vi "PLC Project.vi"() -> ()   [LabVIEW 2022 SP3]
uses:
  <vilib>/MakerHub/LINX/Public/Peripherals/Digital/Digital Read 1 Chan.vi
  <vilib>/MakerHub/LINX/Public/Peripherals/PWM/PWM Set Duty Cycle 1 Chan.vi
  <vilib>/MakerHub/LINX/Public/Peripherals/Digital/Digital Write 1 Chan.vi
  <vilib>/MakerHub/LINX/Public/Peripherals/Digital/Digital Read N Chans.vi
  <vilib>/MakerHub/LINX/Public/Peripherals/Digital/Digital Write N Chans.vi
  <vilib>/MakerHub/LINX/Private/Local IO/LinxDigitalRead.vi
  <vilib>/MakerHub/LINX/Public/Utilities/Check Channel.vi
  <vilib>/MakerHub/LINX/Private/Local IO/LinxDigitalWrite.vi
  <vilib>/MakerHub/LINX/Public/Utilities/Open Serial.vi
  <vilib>/MakerHub/LINX/Private/Utilties/Generate Error.vi
  <vilib>/MakerHub/LINX/Public/Peripherals/PWM/PWM Set Duty Cycle N Chans.vi
  <vilib>/MakerHub/LINX/LMH-LINX.lvlib
  <vilib>/MakerHub/LINX/Public/Sensors/Distance/Ultrasonic/Ultrasonic.lvlib
panel:
  out "Centimeters":dbl
  out "Right":bool
  out "Left":bool
  in  "stop":bool
  in  "PWM signal  (0-255)":dbl
  in  "Input 1":bool
  in  "Input 3":bool
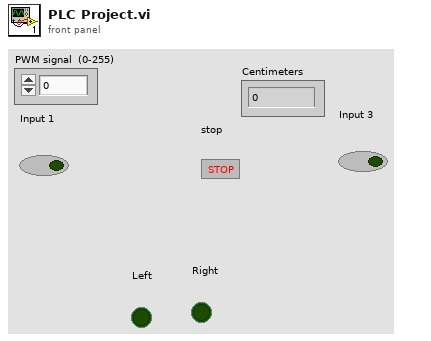
[diagram p1: front panel]
types:
  T1 = typedef "LMH-LINX.lvlib/LINX Ref.ctl" = cluster{"IO":T2, "Interface":T3, "LINX Device Config":T4}
  T2 = typedef "LMH-LINX.lvlib/Platform.ctl" = enum16{"Remote", "Local"}
  T3 = typedef "LMH-LINX.lvlib/Interface.ctl" = enum16{"Serial", "TCP"}
  T4 = typedef "LMH-LINX.lvlib/Device.lvlib/LINX Device Config.ctl" = cluster{"Interface":T3, "COM Port":refnum<visa-resource-name>, "TCP Configuration":T5, "Device Family":u8, "Device ID":u8, "Device Name":string, "TCP Ref":refnum<k5>, "Channels":T6}
  T5 = typedef "LMH-LINX.lvlib/Device.lvlib/TCP Config.ctl" = cluster{"IP Address":string, "Port":u16}
  T6 = typedef "LMH-LINX.lvlib/Channels.ctl" = cluster{"DI":u8[], "DO":u8[], "AI":u8[], "AO":u8[], "PWM":u8[], "QE":u8[], "UART":u8[], "I2C 2":u8[], "SPI":u8[], "CAN":u8[], "Servo":u8[], "AI Ref (V)":dbl, "AI Resolution (Bits)":u8, "AO Ref (V)":dbl, "AO Resolution (Bits)":u8}
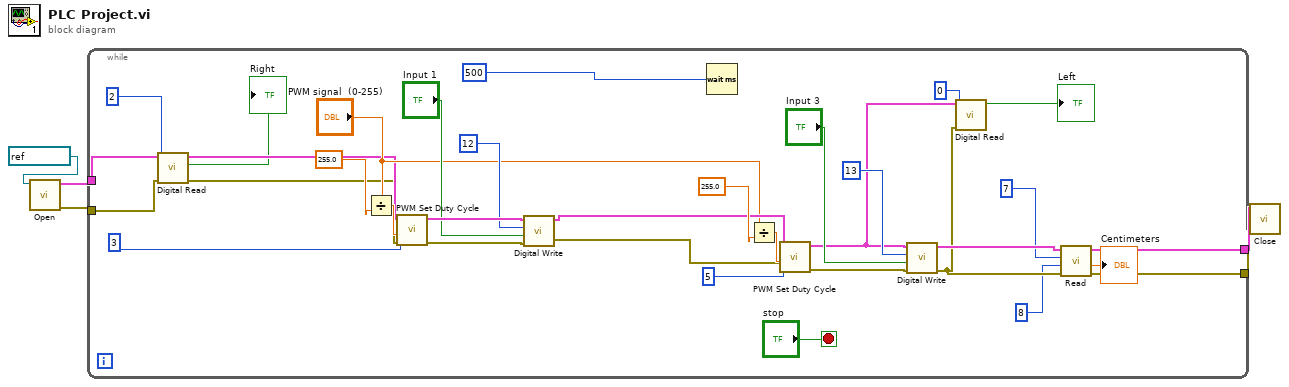
[diagram p0: block diagram]
diagram:
  n1 = call-poly <vilib>:"Open.vi"("Serial Port"=refnum<visa-resource-name> "COM5") -> ("Error Out"=w3:errorcluster, "LINX Resource"=w4:T1)  [unwired: 8 in, 1 out]
  n2 = while {
    tunnel: w4 -> [w21]
    tunnel: w3 -> [w19]
    tunnel: [w10] -> w2
    tunnel: [w9] -> w1
    stop <- "stop" stop-if-true
    n3 = call-poly <vilib>:"Digital Read.vi"("Error In"=w19, "DI Channel"=u8 2, "LINX Resource"=w21) -> ("Error Out"=w17:errorcluster, "DI Value"=→"Right":bool, "LINX Resource"=w18:T1)  [unwired: 6 in]
    n4 = Divide(x="PWM signal  (0-255)", y=255.0) -> (x/y=w35:dbl)
    n5 = call-poly <vilib>:"PWM Set Duty Cycle.vi"("Error In"=w17, "Duty Cycle (0-1)"=w35, "PWM Channel"=u8 3, "LINX Resource"=w18) -> ("Error Out"=w32:errorcluster, "LINX Resource"=w34:T1)  [unwired: 6 in]
    n6 = call-poly <vilib>:"Digital Write.vi"("Error In"=w32, "Output Value"="Input 1", "DO Channel"=u8 12, "LINX Resource"=w34) -> ("Error Out"=w23:errorcluster, "LINX Resource"=w24:T1)  [unwired: 6 in]
    n7 = Wait (ms)(milliseconds to wait=u32 500) -> ()  [unwired: 1 out]
    n8 = Divide(x="PWM signal  (0-255)", y=255.0) -> (x/y=w29:dbl)
    n9 = call-poly <vilib>:"PWM Set Duty Cycle.vi"("Error In"=w23, "Duty Cycle (0-1)"=w29, "PWM Channel"=u8 5, "LINX Resource"=w24) -> ("Error Out"=w27:errorcluster, "LINX Resource"=w16:T1)  [unwired: 6 in]
    n10 = call-poly <vilib>:"Digital Write.vi"("Error In"=w27, "Output Value"="Input 3", "DO Channel"=u8 13, "LINX Resource"=w16) -> ("Error Out"=w13:errorcluster, "LINX Resource"=w14:T1)  [unwired: 6 in]
    n11 = call-poly <vilib>:"Digital Read.vi"("Error In"=w13, "DI Channel"=u8 0, "LINX Resource"=w16) -> ("DI Value"=→"Left":bool)  [unwired: 6 in, 2 out]
    n12 = call <vilib>:"Read.vi"("Error In"=w13, "DO Channel"=u8 8, "DI Channel"=u8 7, "LINX Resource"=w14) -> ("Error Out"=w9:errorcluster, "Centimeters"=→"Centimeters":dbl, "LINX Resource"=w10:T1)  [unwired: 4 in, 1 out]
  }
  n13 = call <vilib>:"Close.vi"("Error In"=w1, "LINX Resource"=w2) -> ()  [unwired: 9 in, 1 out]
